vi "Terminate.vi"(8 "error in (no error)":errorcluster, 11 "Instrument in":refnum<class "DMM.NI.lvclass">) -> (0 "error out":errorcluster, 3 "Instrument out":refnum<class "DMM.NI.lvclass">)   [LabVIEW 2020, in "NI DMM Driver.lvlib" / "DMM.NI.lvclass"]
doc: "Terminate the Instrument.\n\nClose the NI DMM connection."
uses:
  DMM.NI.lvclass
  DMM.NI.lvclass/DMM.NI.ctl
  PPL/HDH.Driver.DMM.lvlibp/DMM Driver.lvclass
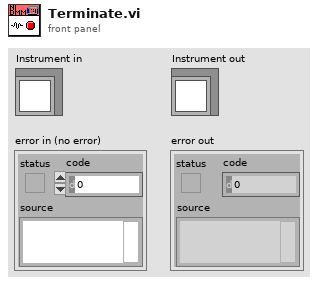
[diagram p1: front panel]
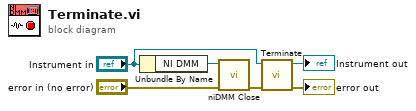
[diagram p0: block diagram]
diagram:
  n1 = Unbundle By Name("Instrument in") -> ("NI DMM"=w3:refnum<k15>)
  n2 = call <instrlib>:"niDMM Close.vi"("error in (no error)"="error in (no error)", "instrument handle"=w3) -> ("error out"=w1:errorcluster)  [unwired: 9 in]
  n3 = call-parent "Terminate.vi"("error in (no error)"=w1, "Instrument in"="Instrument in") -> ("error out"=→"error out":errorcluster, "Instrument out"=→"Instrument out":refnum<class "DMM.NI.lvclass">)  [unwired: 8 in]
